vi "Teleop.vi"(10 "Match Info":T1={"Autonomous Elapsed Seconds"=0.0, "TeleOp Elapsed Seconds"=0.0, "Disabled Elapsed Seconds"=0.0, "Visited Autonomous"=FALSE, "Visited TeleOp"=FALSE, "Visited Disabled"=FALSE, "Autonomous Settings"={"Autonomous Style"=enum."Independent", "VI Refnum"=refnum}}, 11 "Call Context":T2) -> ()   [LabVIEW 2025]
doc: "This VI is called for each TeleOp packet received from the DS where the robot is not disabled. It is often used to read from the joysticks and update I/O or to update setpoints for timed control loops. It should complete and return within 20 milliseconds or it may miss DS packets."
uses:
  <vilib>/Rock Robotics/WPI/DriverStation/WPI_DriverStationDerivedRobotMode.ctl
  <vilib>/Rock Robotics/WPI/DriverStation/WPI_DriverStationMatch Info.ctl
  <vilib>/Rock Robotics/WPI/ThirdParty/REV Robotics/REVLib/Typedef/Spark MAX Control Type.ctl
  <vilib>/Rock Robotics/WPI/ThirdParty/NavX/_TypeDefs/FRIC_navX_DeviceNumbersTypeDef.ctl
  <vilib>/Rock Robotics/WPI/Utilities/WPI_GetSetVariantRefNum.vi
  <vilib>/Rock Robotics/Network Tables/NT Write Boolean Array.vi
  <vilib>/Rock Robotics/Network Tables/NT Write Numeric Array.vi
  <vilib>/Rock Robotics/Network Tables/NT Read Boolean.vi
  <vilib>/Rock Robotics/Network Tables/NT Read Number.vi
  <vilib>/Rock Robotics/Network Tables/NT Write Number.vi
  <vilib>/Rock Robotics/Network Tables/NT Write Variant.vi
panel:
  out "Sample Slider 0":dbl(slide) scale=0.0..5.0
  out "Sample Boolean 1":bool
  out "Sample Boolean 0":bool
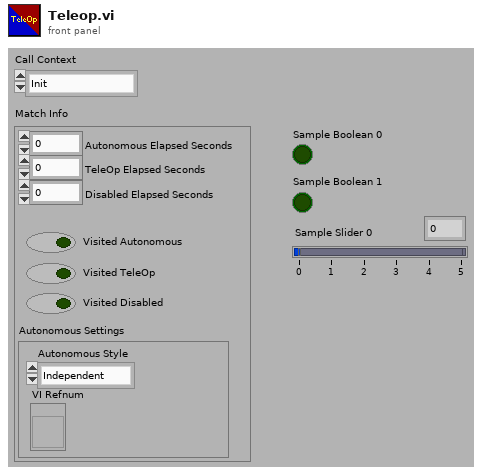
[diagram p1: front panel]
types:
  T1 = typedef "WPI_DriverStationMatch Info.ctl" = cluster{"Autonomous Elapsed Seconds":dbl, "TeleOp Elapsed Seconds":dbl, "Disabled Elapsed Seconds":dbl, "Visited Autonomous":bool, "Visited TeleOp":bool, "Visited Disabled":bool, "Autonomous Settings":cluster{"Autonomous Style":enum16{"Iterative", "Independent"}, "VI Refnum":refnum<vi>}}
  T2 = typedef "WPI_DriverStationDerivedRobotMode.ctl" = enum16{"Init", "Execute", "Stop"}
  T3 = typedef "FRIC_navX_DeviceNumbersTypeDef.ctl" = enum16{"Dev0", "Dev1", "Dev2", "Dev3"}
  T4 = typedef "Spark MAX Control Type.ctl" = enum16{"Percent VBus", "Voltage", "Velocity", "Position", "Smart Motion", "Current", "Smart Velocity", "MAXMotion Position", "MAXMotion Velocity"}
  T5 = cluster{"Yaw":dbl, "Roll":dbl, "Pitch":dbl, "Heading":dbl, "Fused Heading":dbl}
  T6 = cluster{"Rollover":dbl, "Yaw":dbl, "Cont Yaw":dbl}
  T7 = typedef "WPI_JoystickDevRef.ctl" = cluster{"Device":T8}
  T8 = typedef "WPI_JoystickDeviceEnum.ctl" = enum16{"USB 0", "USB 1", "USB 2", "USB 3", "USB 4", "USB 5"}
  T9 = typedef "WPI_ServoDeviceRef.ctl" = cluster{"DeviceStatus":errorcluster, "PWM Channel":T10, "DeadBand":T11}
  T10 = typedef "FPGA_DIOPWMChannel.ctl" = enum8{"PWM 0", "PWM 1", "PWM 2", "PWM 3", "PWM 4", "PWM 5", "PWM 6", "PWM 7", "PWM 8", "PWM 9", "PWM MXP 0", "PWM MXP 1", "PWM MXP 2", "PWM MXP 3", "PWM MXP 4", "PWM MXP 5", "PWM MXP 6", "PWM MXP 7", "PWM MXP 8", "PWM MXP 9", "Invalid"}
  T11 = typedef "WPI_PWMDeadband.ctl" = cluster{"Name":string, "maxPositivePwm":i32, "minPositivePwm":i32, "centerPwm":i32, "maxNegativePwm":i32, "minNegativePwm":i32, "angularRange":u16}
  T12 = typedef "WPI_MotorControlDeviceRef.ctl" = cluster{"DeviceStatus":errorcluster, "Type":T13, "PWM":cluster{"PWM Channel":T10, "DeadBand":T11}, "CAN":cluster{"Device Number":u8, "SetOutput VI Ref":variant, "GetOutput VI Ref":variant, "Enable VI Ref":variant, "Disable VI Ref":variant, "Data":variant}, "Invert":bool, "DIO PWM":cluster{"PWM \"Enable\" Channel":T10, "DIOChannel":T14, "PWM Rate":dbl}}
  T13 = typedef "WPI_MotorControlType.ctl" = enum16{"PWM", "CAN", "DIO PWM"}
  T14 = typedef "FPGA_DIOChannel.ctl" = enum8{"DIO 0", "DIO 1", "DIO 2", "DIO 3", "DIO 4", "DIO 5", "DIO 6", "DIO 7", "DIO 8", "DIO 9", "DIO MXP 0", "DIO MXP 1", "DIO MXP 2", "DIO MXP 3", "DIO MXP 4", "DIO MXP 5", "DIO MXP 6", "DIO MXP 7", "DIO MXP 8", "DIO MXP 9", "DIO MXP 10", "DIO MXP 11", "DIO MXP 12", "DIO MXP 13", "DIO MXP 14", "DIO MXP 15", "SPI Port CS1", "SPI Port CS2", "SPI Port CS3", "SPI Port MISO", "SPI Port MOSI", "Invalid"}
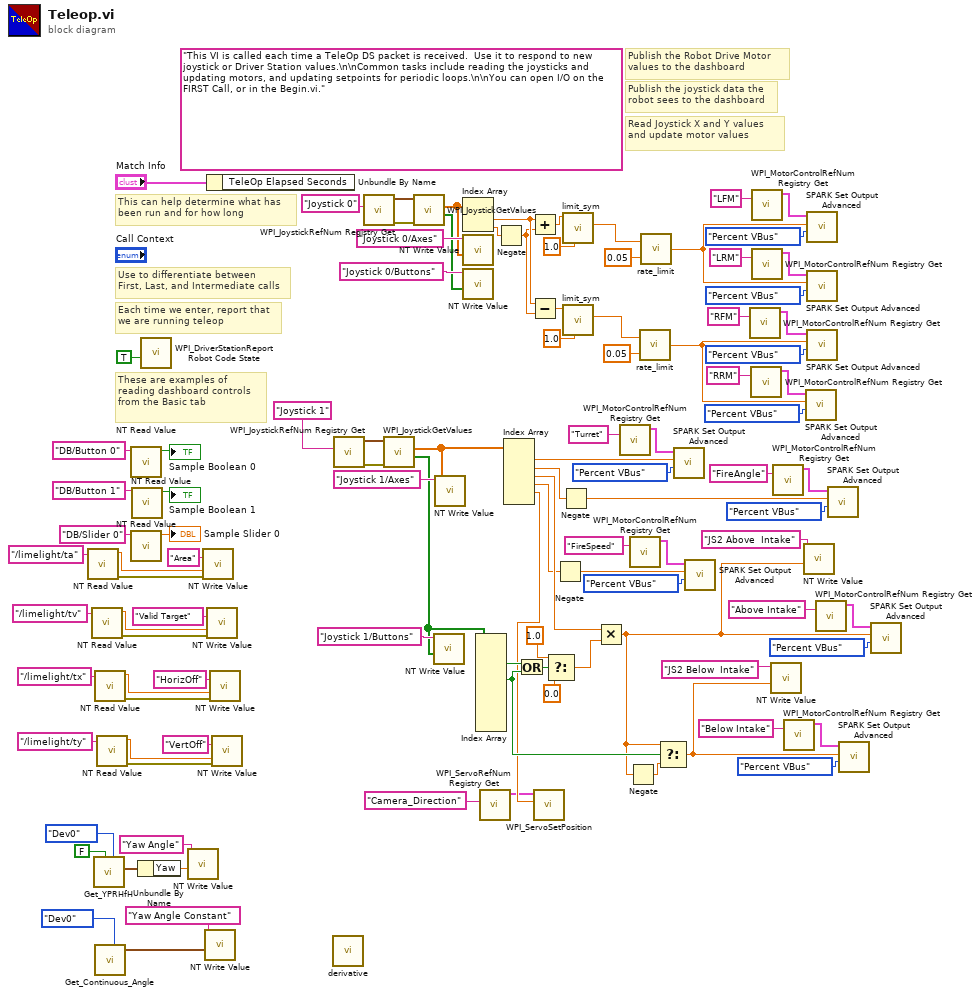
[diagram p0: block diagram]
diagram:
  (unwired) "This VI is called each time a TeleOp DS packet is received.  Use it to respond to new joystick or Driver Station values.\n\nCommon tasks include reading the joysticks and updating motors, and updating setpoints for periodic loops.\n\nYou can open I/O on the FIRST Call, or in the Begin.vi."
  # "These are examples of reading dashboard controls from the Basic tab"
  # "Publish the Robot Drive Motor\nvalues to the dashboard"
  # "Publish the joystick data the\nrobot sees to the dashboard"
  # "Each time we enter, report that\nwe are running teleop"
  # "Use to differentiate between\nFirst, Last, and Intermediate calls"
  # "This can help determine what has\nbeen run and for how long"
  # "Read Joystick X and Y values and update motor values"
  n1 = call-poly <vilib>:"NT Read Value.vi"("name"="/limelight/ta") -> ("error out"=w55:errorcluster, "value"=w56:dbl)  [unwired: 8 in, 1 out]
  n2 = call-poly <vilib>:"NT Read Value.vi"("name"="/limelight/tv") -> ("error out"=w60:errorcluster, "value"=w61:dbl)  [unwired: 8 in, 1 out]
  n3 = call <vilib>:"Get_YPRHfH.vi"("Device Number"=FRIC_navX_DeviceNumbersTypeDef."Dev0", "Update"=FALSE) -> ("YRPHfH"=w16:T5)  [unwired: 9 in]
  n4 = call-poly <vilib>:"NT Read Value.vi"("name"="/limelight/tx") -> ("error out"=w53:errorcluster, "value"=w54:dbl)  [unwired: 8 in, 1 out]
  n5 = call <vilib>:"Get_Continuous_Angle.vi"("Device Number"=FRIC_navX_DeviceNumbersTypeDef."Dev0") -> ("Continuous Angle"=w1:T6)  [unwired: 10 in]
  n6 = call-poly <vilib>:"NT Read Value.vi"("name"="/limelight/ty") -> ("error out"=w52:errorcluster, "value"=w51:dbl)  [unwired: 8 in, 1 out]
  n7 = call-poly <vilib>:"NT Read Value.vi"("name"="DB/Button 0" ("refnum name")) -> ("value"=→"Sample Boolean 0":bool)  [unwired: 8 in, 2 out]
  n8 = call-poly <vilib>:"NT Read Value.vi"("name"="DB/Slider 0" ("refnum name")) -> ("value"=→"Sample Slider 0":dbl)  [unwired: 8 in, 2 out]
  n9 = call-poly <vilib>:"NT Read Value.vi"("name"="DB/Button 1" ("refnum name")) -> ("value"=→"Sample Boolean 1":bool)  [unwired: 8 in, 2 out]
  n10 = Unbundle By Name(w16) -> ("Yaw"=w14:dbl)
  n11 = call <vilib>:"WPI_DriverStationReport Robot Code State.vi"("TeleOp"=TRUE ("Autonomous")) -> ()  [unwired: 10 in, 1 out]
  n12 = call-poly <vilib>:"NT Write Value.vi"("value"=w14, "name"="Yaw Angle") -> ()  [unwired: 9 in, 1 out]
  n13 = call-poly <vilib>:"NT Write Value.vi"("error in"=w55, "value"=w56, "name"="Area") -> ()  [unwired: 8 in, 1 out]
  n14 = call-poly <vilib>:"NT Write Value.vi"("variant"=w1, "name"="Yaw Angle Constant") -> ()  [unwired: 9 in, 1 out]
  n15 = Unbundle By Name("Match Info") -> ()  [unwired: 1 out]
  n16 = call-poly <vilib>:"NT Write Value.vi"("error in"=w60, "value"=w61, "name"="Valid Target") -> ()  [unwired: 8 in, 1 out]
  n17 = call-poly <vilib>:"NT Write Value.vi"("error in"=w53, "value"=w54, "name"="HorizOff") -> ()  [unwired: 8 in, 1 out]
  n18 = call-poly <vilib>:"NT Write Value.vi"("error in"=w52, "value"=w51, "name"="VertOff") -> ()  [unwired: 8 in, 1 out]
  n19 = call "derivative.vi"() -> ()  [unwired: 4 in, 1 out]
  n20 = call <vilib>:"WPI_JoystickRefNum Registry Get.vi"("refnum name"="Joystick 1") -> ("error out"=w46:errorcluster, "JoystickDevRef"=w73:T7)  [unwired: 1 in, 8 out]
  n21 = call <vilib>:"WPI_JoystickRefNum Registry Get.vi"("refnum name"="Joystick 0") -> ("error out"=w45:errorcluster, "JoystickDevRef"=w104:T7)  [unwired: 1 in, 8 out]
  n22 = call <vilib>:"WPI_JoystickGetValues.vi"("error in (no error)"=w46, "JoystickDevRef"=w73) -> ("Buttons"=w44:bool[], "Axes"=w70:dbl[])  [unwired: 5 in, 3 out]
  n23 = call <vilib>:"WPI_JoystickGetValues.vi"("error in (no error)"=w45, "JoystickDevRef"=w104) -> ("Buttons"=w99:bool[], "Axes"=w100:dbl[])  [unwired: 5 in, 3 out]
  n24 = call-poly <vilib>:"NT Write Value.vi"("value"=w44, "name"="Joystick 1/Buttons" ("Name")) -> ()  [unwired: 9 in, 1 out]
  n25 = call-poly <vilib>:"NT Write Value.vi"("value"=w70, "name"="Joystick 1/Axes" ("Name")) -> ()  [unwired: 9 in, 1 out]
  n26 = Index Array(array=w100) -> (element #1=w77:dbl, element #2=w76:dbl)  [unwired: 2 in]
  n27 = call-poly <vilib>:"NT Write Value.vi"("value"=w100, "name"="Joystick 0/Axes" ("Name")) -> ()  [unwired: 9 in, 1 out]
  n28 = call-poly <vilib>:"NT Write Value.vi"("value"=w99, "name"="Joystick 0/Buttons" ("Name")) -> ()  [unwired: 9 in, 1 out]
  n29 = Index Array(array=w44) -> (element #2=w39:bool, element #4=w30:bool)  [unwired: 10 in, 8 out]
  n30 = call <vilib>:"WPI_ServoRefNum Registry Get.vi"("refnum name"="Camera_Direction") -> ("ServoDeviceRef"=w10:T9)  [unwired: 9 in, 1 out]
  n31 = Negate(x=w76) -> (-x=w75:dbl)
  n32 = Index Array(array=w70) -> (element #1=w34:dbl, element #2=w20:dbl, element #3=w32:dbl, element #4=w24:dbl, element #5=w11:dbl)  [unwired: 6 in, 1 out]
  n33 = Or(x=w39, y=w30) -> (x .or. y?=w38:bool)
  n34 = Add(x=w77, y=w75) -> (x+y=w81:dbl)
  n35 = Subtract(x=w77, y=w75) -> (x-y=w80:dbl)
  n36 = call <vilib>:"WPI_ServoSetPosition.vi"("Position"=w11, "ServoDeviceRef"=w10) -> ()  [unwired: 8 in, 2 out]
  n37 = Select(t=1.0, s=w38, f=0.0 ("t")) -> (s? t:f=w42:dbl)
  n38 = Negate(x=w24) -> (-x=w25:dbl)
  n39 = Negate(x=w20) -> (-x=w19:dbl)
  n40 = call "limit_sym.vi"("Limit"=1.0, "Input"=w81) -> ("Output"=w7:dbl)  [unwired: 9 in]
  n41 = call "limit_sym.vi"("Limit"=1.0, "Input"=w80) -> ("Output"=w5:dbl)  [unwired: 9 in]
  n42 = Multiply(x=w32, y=w42) -> (x*y=w29:dbl)
  n43 = call <vilib>:"WPI_MotorControlRefNum Registry Get.vi"("refnum name"="Turret") -> ("MotorControlDevRef"=w35:T12)  [unwired: 9 in, 1 out]
  n44 = Negate(x=w29) -> (-x=w41:dbl)
  n45 = call <vilib>:"WPI_MotorControlRefNum Registry Get.vi"("refnum name"="FireSpeed") -> ("MotorControlDevRef"=w28:T12)  [unwired: 9 in, 1 out]
  n46 = call "rate_limit.vi"("Rate Limit"=0.05, "In"=w5) -> ("Out"=w4:dbl)
  n47 = call "rate_limit.vi"("Rate Limit"=0.05, "In"=w7) -> ("Out"=w6:dbl)
  n48 = Select(t=w29, s=w30, f=w41) -> (s? t:f=w33:dbl)
  n49 = call <vilib>:"SPARK Set Output Advanced.vi"("Control Mode"=Spark_MAX_Control_Type."Percent VBus", "Setpoint"=w34, "MotorControlDevRef"=w35) -> ()  [unwired: 7 in, 2 out]
  n50 = call <vilib>:"SPARK Set Output Advanced.vi"("Control Mode"=Spark_MAX_Control_Type."Percent VBus", "Setpoint"=w25, "MotorControlDevRef"=w28) -> ()  [unwired: 7 in, 2 out]
  n51 = call <vilib>:"WPI_MotorControlRefNum Registry Get.vi"("refnum name"="RFM") -> ("MotorControlDevRef"=w90:T12)  [unwired: 9 in, 1 out]
  n52 = call <vilib>:"WPI_MotorControlRefNum Registry Get.vi"("refnum name"="RRM") -> ("MotorControlDevRef"=w87:T12)  [unwired: 9 in, 1 out]
  n53 = call <vilib>:"WPI_MotorControlRefNum Registry Get.vi"("refnum name"="LFM") -> ("MotorControlDevRef"=w85:T12)  [unwired: 9 in, 1 out]
  n54 = call <vilib>:"WPI_MotorControlRefNum Registry Get.vi"("refnum name"="LRM") -> ("MotorControlDevRef"=w93:T12)  [unwired: 9 in, 1 out]
  n55 = call-poly <vilib>:"NT Write Value.vi"("value"=w33, "name"="JS2 Below  Intake") -> ()  [unwired: 9 in, 1 out]
  n56 = call <vilib>:"WPI_MotorControlRefNum Registry Get.vi"("refnum name"="FireAngle") -> ("MotorControlDevRef"=w21:T12)  [unwired: 9 in, 1 out]
  n57 = call <vilib>:"WPI_MotorControlRefNum Registry Get.vi"("refnum name"="Below Intake") -> ("MotorControlDevRef"=w69:T12)  [unwired: 9 in, 1 out]
  n58 = call-poly <vilib>:"NT Write Value.vi"("value"=w29, "name"="JS2 Above  Intake") -> ()  [unwired: 9 in, 1 out]
  n59 = call <vilib>:"SPARK Set Output Advanced.vi"("Control Mode"=Spark_MAX_Control_Type."Percent VBus", "Setpoint"=w4, "MotorControlDevRef"=w87) -> ()  [unwired: 7 in, 2 out]
  n60 = call <vilib>:"SPARK Set Output Advanced.vi"("Control Mode"=Spark_MAX_Control_Type."Percent VBus", "Setpoint"=w6, "MotorControlDevRef"=w85) -> ()  [unwired: 7 in, 2 out]
  n61 = call <vilib>:"SPARK Set Output Advanced.vi"("Control Mode"=Spark_MAX_Control_Type."Percent VBus", "Setpoint"=w6, "MotorControlDevRef"=w93) -> ()  [unwired: 7 in, 2 out]
  n62 = call <vilib>:"SPARK Set Output Advanced.vi"("Control Mode"=Spark_MAX_Control_Type."Percent VBus", "Setpoint"=w4, "MotorControlDevRef"=w90) -> ()  [unwired: 7 in, 2 out]
  n63 = call <vilib>:"WPI_MotorControlRefNum Registry Get.vi"("refnum name"="Above Intake") -> ("MotorControlDevRef"=w50:T12)  [unwired: 9 in, 1 out]
  n64 = call <vilib>:"SPARK Set Output Advanced.vi"("Control Mode"=Spark_MAX_Control_Type."Percent VBus", "Setpoint"=w19, "MotorControlDevRef"=w21) -> ()  [unwired: 7 in, 2 out]
  n65 = call <vilib>:"SPARK Set Output Advanced.vi"("Control Mode"=Spark_MAX_Control_Type."Percent VBus", "Setpoint"=w33, "MotorControlDevRef"=w69) -> ()  [unwired: 7 in, 2 out]
  n66 = call <vilib>:"SPARK Set Output Advanced.vi"("Control Mode"=Spark_MAX_Control_Type."Percent VBus", "Setpoint"=w29, "MotorControlDevRef"=w50) -> ()  [unwired: 7 in, 2 out]
